vi "Write Text_Format.vi"(8 "error in (no error)":errorcluster caption="에러 입력(에러 없음)", 10 "Text_Format":T1={"TXT_Radix"=enum."HEX", "TXT_Prefix"=TRUE, "TXT_Delimiter"="\r\n", "TXT_End of LIne"=enum."EOL (\\r\\n)", "TXT_EOL+Delimiter"=TRUE, "TXT_Number per Line"=1} {"TXT_Number per Line" min=1 max=100}, 11 "Text File 입력":refnum<class "Text File.lvclass">) -> (0 "error out":errorcluster caption="에러 출력", 3 "Text File 출력":refnum<class "Text File.lvclass">)   [LabVIEW 2020, in "Text File.lvclass"]
uses:
  Text File.lvclass
  Text File.lvclass/Text File.ctl
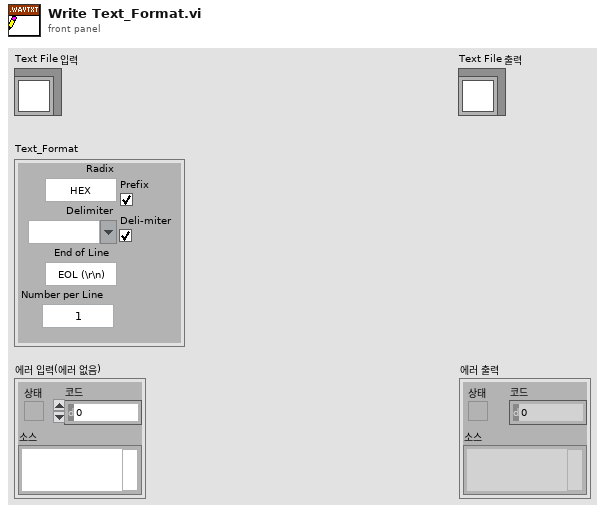
[diagram p1: front panel]
types:
  T1 = cluster{"TXT_Radix":enum16{"BIN", "DEC", "HEX"}, "TXT_Prefix":bool, "TXT_Delimiter":string, "TXT_End of LIne":enum16{"EOL (\\r\\n)", "LF (\\n)"}, "TXT_EOL+Delimiter":bool, "TXT_Number per Line":i32}
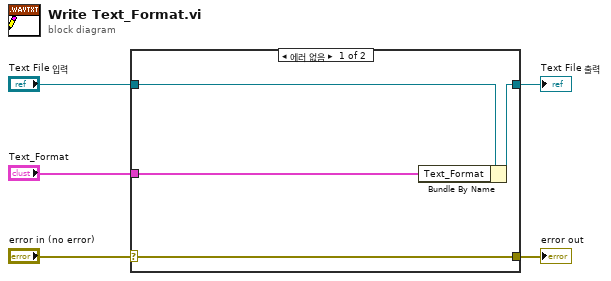
[diagram p0: block diagram]
diagram:
  n1 = case shown="에러 없음" "error in (no error)" {
    selector: "error in (no error)" -> [w9 w10]
    tunnel: [w9 w10] -> w4
    tunnel: [w7 w11] -> w2
    tunnel: "Text File 입력" -> [w8 w11]
    tunnel: "Text_Format" -> [w6 _]
    frame No Error {
      n2 = Bundle By Name(cluster=w8, "Text_Format"=w6) -> (w7:refnum<class "Text File.lvclass">)
    }
    frame Error {
    }
  }
  "error out" <- w4
  "Text File 출력" <- w2
